vi "myo_unlock.vi"(6 "Connection Status":T2={"MAC Address"="", "cnx handle"=0, "cnx flags"=0, "Address Type"=125, "Connection Interval (ms)"=125, "Timeout(ms)"=125, "Latency"=0, "bonding handle"=0} {"Address Type" items=["Public", "Random"]}, 8 "error in (no error)":errorcluster, 9 "Unlock types(Relock)":T1 items=["Re-lock", "Unlock (timeout)", "Unlock"], 10 "Handle table":string[][](array[string]), 11 "VISA Refnum in":refnum<visa-resource-name>) -> (0 "error out":errorcluster, 3 "VISA Refnum out":refnum<visa-resource-name>)   [LabVIEW 2013]
uses:
  code/labview/bluetooth_le/bluegiga/type_def/connection_status_bundle.ctl
  code/labview/bluetooth_le/bluegiga/type_def/address_type.ctl
  type_def/unlock_types.ctl
  code/labview/bluetooth_le/bluegiga/functions/ble_write_by_service_characteristic_uint8array.vi
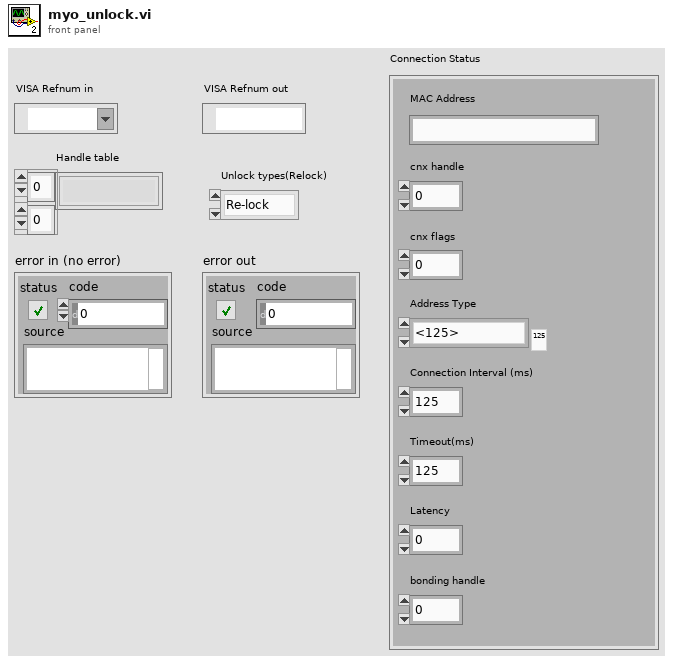
[diagram p1: front panel]
types:
  T1 = typedef "unlock_types.ctl" = u8
  T2 = typedef "connection_status_bundle.ctl" = cluster{"MAC Address":string, "cnx handle":u8, "cnx flags":u8, "Address Type":T3, "Connection Interval (ms)":u16, "Timeout(ms)":u16, "Latency":u16, "bonding handle":u8}
  T3 = typedef "address_type.ctl" = u8
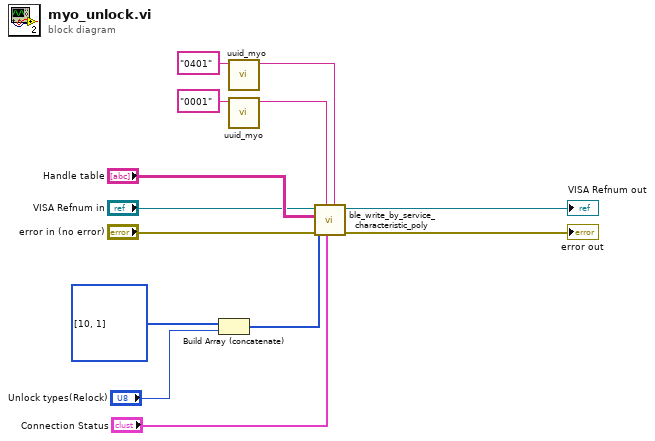
[diagram p0: block diagram]
diagram:
  n1 = Build Array (concatenate)(u8[] [10, 1] ("data"), "Unlock types(Relock)") -> (w3:T1[])
  n2 = call "uuid_myo.vi"("MYO  UUID (16bits)"="0401") -> ("full UUID"=w7:string)  [unwired: 10 in]
  n3 = call "uuid_myo.vi"("MYO  UUID (16bits)"="0001") -> ("full UUID"=w8:string)  [unwired: 10 in]
  n4 = call-poly "ble_write_by_service_characteristic_poly.vi"("Characteristic UUID"=w7, "Connection Status"="Connection Status", "Service UUID"=w8, "error in (no error)"="error in (no error)", "data"=w3, "Handle table"="Handle table", "COM Bluegiga in"="VISA Refnum in") -> ("error out"=→"error out":errorcluster, "COM Bluegiga out"=→"VISA Refnum out":refnum<visa-resource-name>)  [unwired: 3 in]
